vi "FV_conv_step_and_turn.vi"(6 "valve_type":enum16{"Run", "Bypass"}(ring), 7 "backlash_corr":bool caption="Backlash Correction", 8 "turn_in_pre":dbl, 9 "turn_in":dbl, 10 "step_in_pre":i32, 11 "step_in":i32) -> (0 "step_corr_for_step_out":i32, 1 "step_out":i32, 2 "step_corr_for_turn_out":i32, 3 "turn_out":dbl)   [LabVIEW 2019]
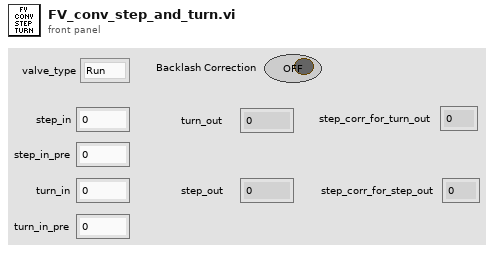
[diagram p1: front panel]
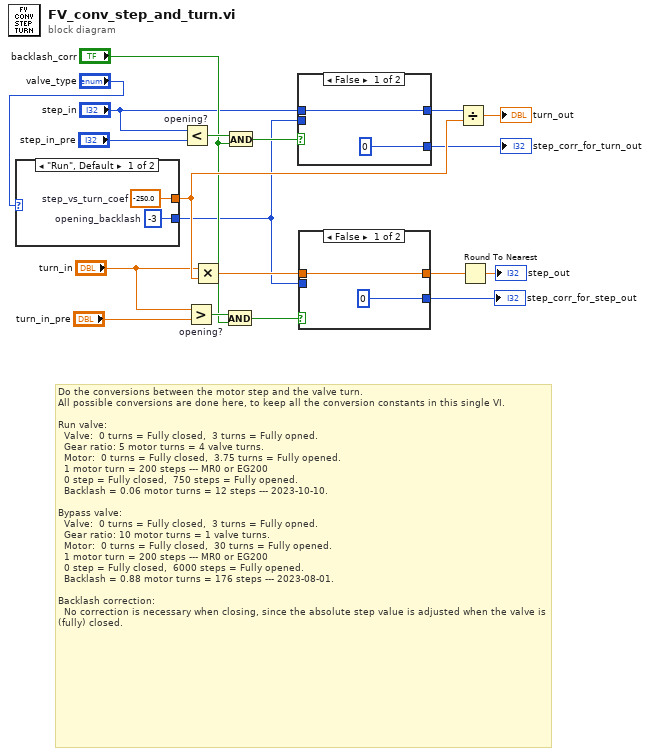
[diagram p0: block diagram]
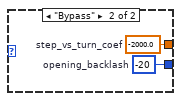
[diagram p2: hidden frame]
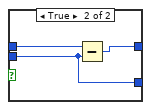
[diagram p3: hidden frame]
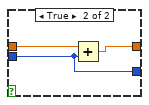
[diagram p4: hidden frame]
diagram:
  # "Do the conversions between the motor step and the valve turn.\nAll possible conversions are done here, to keep all the conversion constants in this single VI.\n\nRun valve:\n  Valve:  0 turns = Fully closed,  3 turns = Fully opned.\n  Gear ratio: 5 motor turns = 4 valve turns.\n  Motor:  0 turns = Fully closed,  3.75 turns = Fully opened.\n  1 motor turn = 200 steps --- MR0 or EG200\n  0 step = Fully closed,  750 steps = Fully opened.\n  Backlash = 0.06 motor turns = 12 steps --- 2023-10-10. \n\nBypass valve:\n  Valve:  0 turns = Fully closed,  3 turns = Fully opned.\n  Gear ratio: 10 motor turns = 1 valve turns.\n  Motor:  0 turns = Fully closed,  30 turns = Fully opened.\n  1 motor turn = 200 steps --- MR0 or EG200\n  0 step = Fully closed,  6000 steps = Fully opened.\n  Backlash = 0.88 motor turns = 176 steps --- 2023-08-01.\n\nBacklash correction:\n  No correction is necessary when closing, since the absolute step value is adjusted when the valve is (fully) closed."
  n1 = case shown="\"Run\", Default" "valve_type" {
    tunnel: [w21 w23] -> w18
    tunnel: [w20 w22] -> w4
    frame "Run", Default {
      w20 = -3  # opening_backlash
      w21 = -250.0  # step_vs_turn_coef
    }
    frame "Bypass" {
      w22 = -20  # opening_backlash
      w23 = -2000.0  # step_vs_turn_coef
    }
  }
  n2 = Less? "opening?"(x="step_in", y="step_in_pre") -> (x < y?=w9:bool)
  n3 = Greater? "opening?"(x="turn_in", y="turn_in_pre") -> (0:w14:bool)
  n4 = Multiply(x="turn_in", y=w18) -> (x*y=w12:dbl)
  n5 = And(x=w14, y="backlash_corr") -> (x .and. y?=w13:bool)
  n6 = And(x=w9, y="backlash_corr") -> (x .and. y?=w7:bool)
  n7 = case shown="False" w7 {
    tunnel: [w25 w27] -> w6
    tunnel: "step_in" -> [w25 w28]
    tunnel: w4 -> [_ w26]
    tunnel: [0 ("opening_backlash") w26] -> w2
    frame False {
    }
    frame True {
      n8 = Subtract(x=w28, y=w26) -> (x-y=w27:i32)
    }
  }
  "step_corr_for_turn_out" <- w2
  n9 = case shown="False" w13 {
    tunnel: w12 -> [w30 w32]
    tunnel: [w30 w33] -> w11
    tunnel: [0 ("step_corr") w31] -> w3
    tunnel: w4 -> [_ w31]
    frame False {
    }
    frame True {
      n10 = Add(x=w32, y=w31) -> (x+y=w33:dbl)
    }
  }
  "step_corr_for_step_out" <- w3
  n11 = Divide(x=w6, y=w18) -> (x/y=→"turn_out":dbl)
  n12 = Round To Nearest(number=w11) -> (nearest integer value=→"step_out":dbl)
